vi "addDoubleElement.vi"(7 "Name":string, 8 "error in (no error)":errorcluster, 9 "Value":dbl, 10 "Replace? (false)":bool, 11 "tBSONDocument in":refnum<class "tBSONDocument.lvclass">) -> (0 "error out":errorcluster, 3 "tBSONDocument out":refnum<class "tBSONDocument.lvclass">)   [LabVIEW 2013, in "BSON.lvlib" / "tBSONDocument.lvclass"]
doc: "Adds a double to a BSON document."
uses:
  tBSONDocument.lvclass
  BSONElements/tBSONDouble/tBSONDouble.lvclass
  tBSONElement/tBSONElement.lvclass
  tBSONElement/setName.vi
  BSONElements/tBSONDouble/setValue.vi
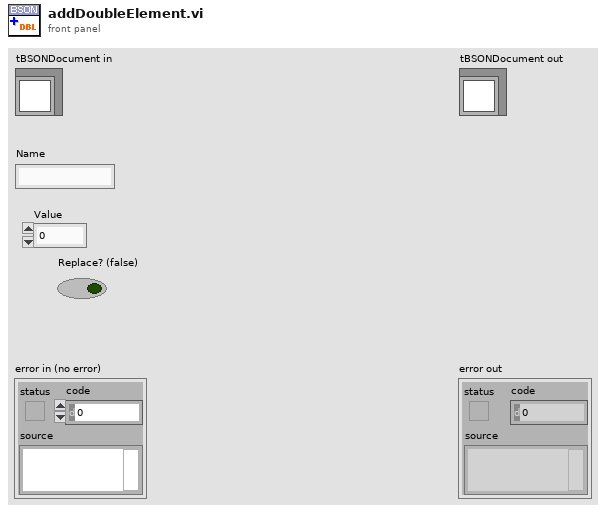
[diagram p1: front panel]
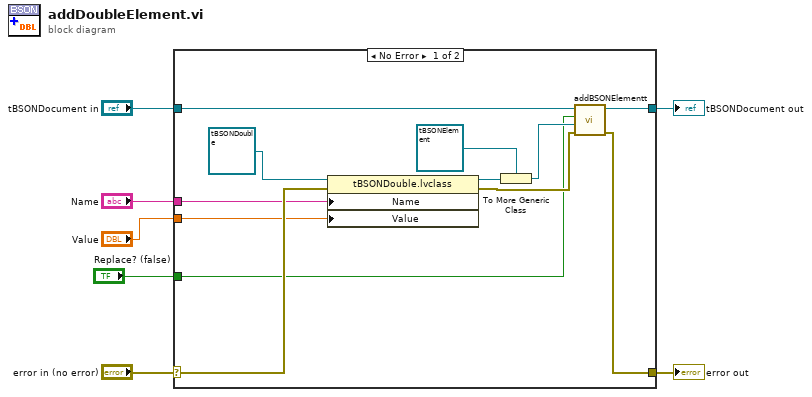
[diagram p0: block diagram]
diagram:
  n1 = case shown="No Error" "error in (no error)" {
    selector: "error in (no error)" -> [w19 w21]
    tunnel: [w9 w21] -> w6
    tunnel: [w10 w20] -> w4
    tunnel: "tBSONDocument in" -> [w13 w20]
    tunnel: "Name" -> [w17 _]
    tunnel: "Value" -> [w16 _]
    tunnel: "Replace? (false)" -> [w8 _]
    frame No Error {
      n2 = property class="tBSONDouble.lvclass"(reference=refnum<class "tBSONDouble.lvclass"> refnum ("BSON.lvlib:tBSONDouble.lvclass"), error in=w19, "Name"=w17, "Value"=w16) -> (reference out=w15:refnum<class "tBSONDouble.lvclass">, error out=w12:errorcluster)
      n3 = To More Generic Class(target class=refnum<class "tBSONElement.lvclass"> refnum ("BSON.lvlib:tBSONElement.lvclass"), reference=w15) -> (generic class reference=w11:refnum<class "tBSONElement.lvclass">)
      n4 = call "addBSONElementt.vi"("error in (no error)"=w12, "Element"=w11, "Replace? (false)"=w8, "tBSONDocument in"=w13) -> ("error out"=w9:errorcluster, "tBSONDocument out"=w10:refnum<class "tBSONDocument.lvclass">)  [unwired: 6 in]
    }
    frame Error {
    }
  }
  "error out" <- w6
  "tBSONDocument out" <- w4
